vi "AutoFeedForwardConversion.vi"(2 "Planned Rotational Velocity (deg/s)":dbl, 3 "Planned Ground Velocity (in/s)":dbl) -> (0 "Equivalent Rotation Joystick Command (ul)":dbl, 1 "Equivalent Strafe Joystick Command (ul)":dbl)   [LabVIEW 2020]
doc: "Converts the feed-forward ground velocity from inches/sec to a unitless drive command and the feed-forward rotational velocity from degrees/sec to a unitless drive command. This VI is intended for use with the FRC 4265 Autonomous Path Planner and the pure-pursuit algorithm."
uses:
  GlobalDrivebase.vi
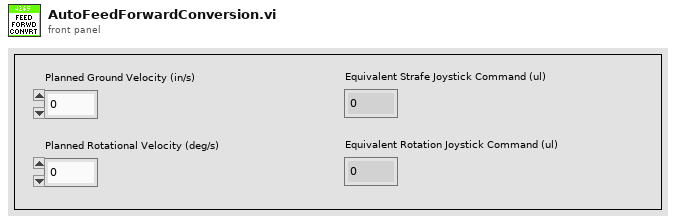
[diagram p1: front panel]
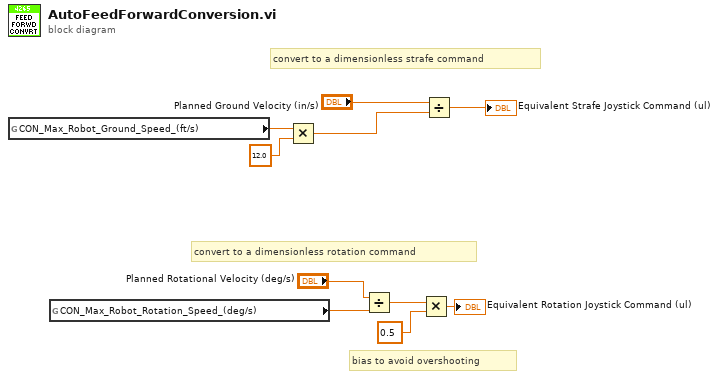
[diagram p0: block diagram]
diagram:
  # "bias to avoid overshooting"
  # "convert to a dimensionless rotation command"
  # "convert to a dimensionless strafe command"
  n1 = global read "GlobalDrivebase.vi" "CON_Max_Robot_Ground_Speed_(ft/s)"() -> (w2:dbl)
  n2 = global read "GlobalDrivebase.vi" "CON_Max_Robot_Rotation_Speed_(deg/s)"() -> (w1:dbl)
  n3 = Multiply(x=w2, y=12.0) -> (x*y=w8:dbl)
  n4 = Divide(x="Planned Rotational Velocity (deg/s)", y=w1) -> (x/y=w4:dbl)
  n5 = Multiply(x=w4, y=0.5 ("Rotation Feed Forward Suppression")) -> (x*y=→"Equivalent Rotation Joystick Command (ul)":dbl)
  n6 = Divide(x="Planned Ground Velocity (in/s)", y=w8) -> (x/y=→"Equivalent Strafe Joystick Command (ul)":dbl)
